vi "Reason_Type.vi"(3 "Reason Type":T1) -> (0 "Break|Bookout":string, 1 "Hint":string)   [LabVIEW 2020]
uses:
  Controls/Loss_type.ctl
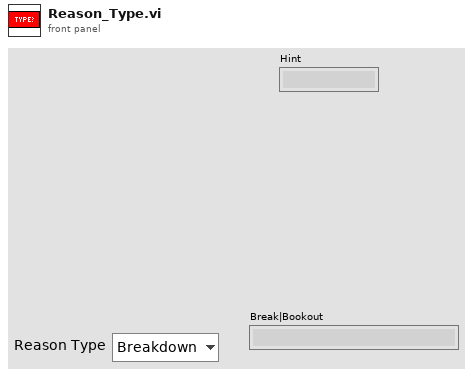
[diagram p1: front panel]
types:
  T1 = typedef "Loss_type.ctl" = enum16{"Breakdown", "Bookout"}
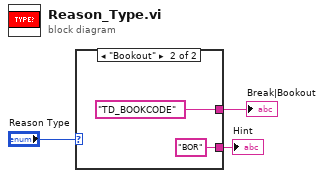
[diagram p0: block diagram]
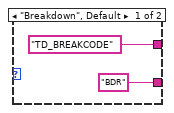
[diagram p2: hidden frame]
diagram:
  n1 = case shown="\"Bookout\"" "Reason Type" {
    tunnel: ["TD_BREAKCODE" ("Break|Bookout") "TD_BOOKCODE" ("Break|Bookout")] -> w2
    tunnel: ["BDR" ("Break|Bookout") "BOR" ("Break|Bookout")] -> w1
    frame "Breakdown", Default {
    }
    frame "Bookout" {
    }
  }
  "Break|Bookout" <- w2
  "Hint" <- w1
